vi "Get Channel Info.vi"(8 "error in (no error)":errorcluster, 11 "FPGA Personality File Path":path) -> (0 "error out":errorcluster, 2 "Channel Info":string[][](array[string]), 3 "Duplicated FPGA Personality File Path":path)   [LabVIEW 2021, in "Personality.lvlib"]
doc: "Gets all channal information from the specified FPGA personality file."
uses:
  <vilib>/myRIO/Common/FPGA Personality Framework/Personality.lvlib
  <vilib>/xml/Load XML File.vi
  <vilib>/xml/Close Reference(Node).vi
  <vilib>/xml/NI_XML.lvlib
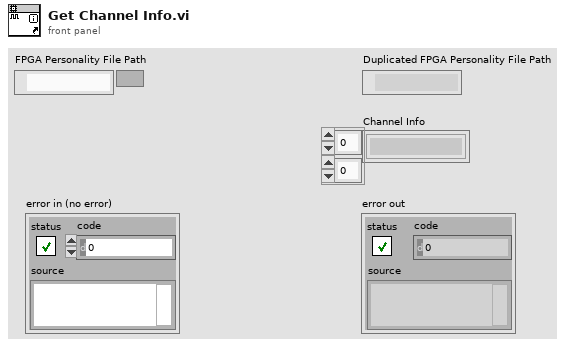
[diagram p1: front panel]
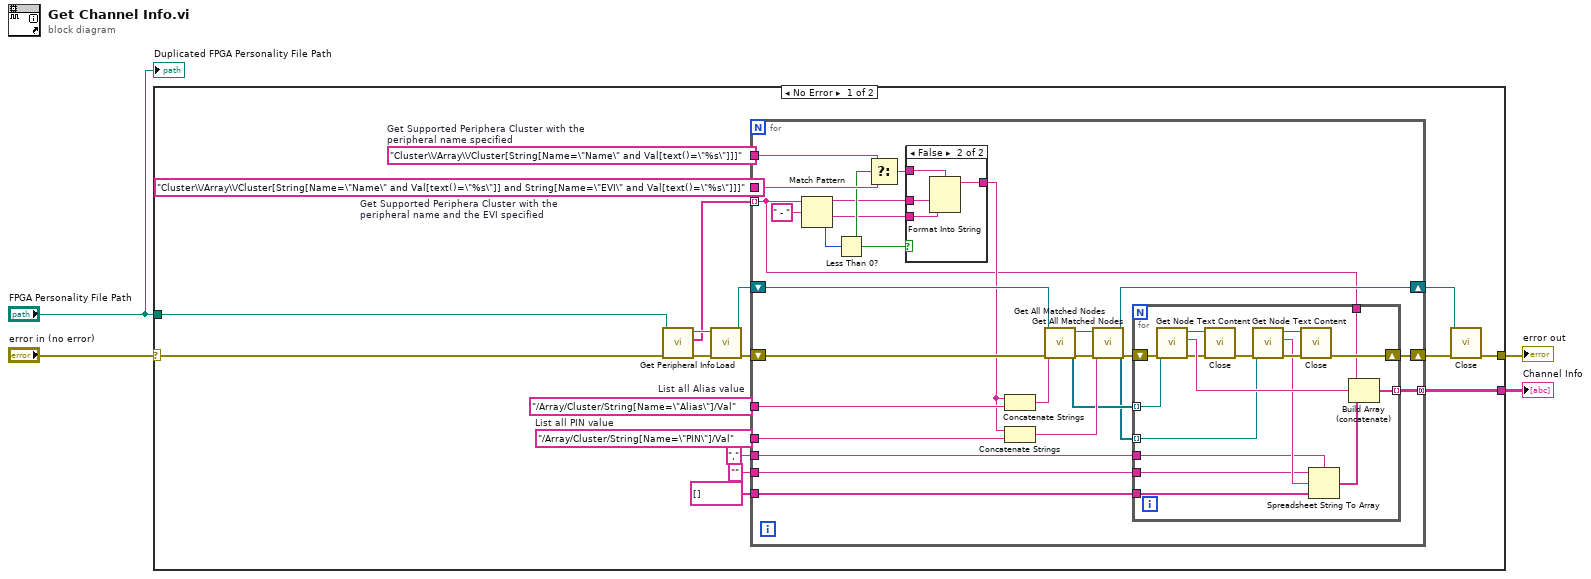
[diagram p0: block diagram]
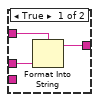
[diagram p2: hidden frame]
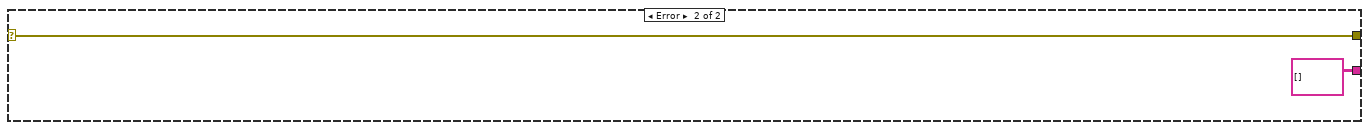
[diagram p3: hidden frame]
diagram:
  n1 = case shown="No Error" "error in (no error)" {
    selector: "error in (no error)" -> [w22 w75]
    tunnel: [w21 w75] -> w3
    tunnel: "FPGA Personality File Path" -> [w20 _]
    tunnel: [w5 string[][] []] -> w1
    frame No Error {
      w9 = "/Array/Cluster/String[Name=\"PIN\"]/Val"  # List all PIN value
      w10 = "/Array/Cluster/String[Name=\"Alias\"]/Val"  # List all Alias value
      w11 = "Cluster\\/Array\\/Cluster[String[Name=\"Name\" and Val[text()=\"%s\"]]]"  # Get Supported Periphera Cluster with the peripheral name specified
      w18 = "Cluster\\/Array\\/Cluster[String[Name=\"Name\" and Val[text()=\"%s\"]] and String[Name=\"EVI\" and Val[text()=\"%s\"]]]"  # Get Supported Periphera Cluster with the peripheral name and the EVI specified
      n2 = call <vilib>:"Get Peripheral Info.vi"("error in (no error)"=w22, "FPGA Personality File Path"=w20) -> ("error out"=w15:errorcluster, "Supported Peripherals"=w12:string[], "Duplicated FPGA Personality File Path"=w14:path)  [unwired: 6 in, 1 out]
      n3 = call-poly <vilib>:"Load.vi"("path to XML document"=w14, "error in (no error)"=w15) -> ("DOM document out"=w16:refnum<k20>, "error out"=w13:errorcluster)  [unwired: 11 in, 1 out]
      n4 = for {
        tunnel: w18 -> [w46]
        shift-right: [w25] -> w19
        shift-left: w13 -> [w49]
        shift-right: [w33] -> w17
        shift-left: w16 -> [w48]
        tunnel: w12 -> [w26] mode=indexing
        tunnel: w11 -> [w45]
        tunnel: w10 -> [w40]
        tunnel: w9 -> [w39]
        tunnel: "," ("delimiter (Tab)") -> [w29]
        tunnel: "" ("format string") -> [w28]
        tunnel: string[] [] -> [w27]
        tunnel: [w24] -> w5 mode=concatenating
        n5 = Match Pattern(string=w26, regular expression=" - ") -> (before substring=w42:string, after substring=w43:string, offset past match=w23:i32)  [unwired: 1 in, 1 out]
        n6 = Less Than 0?(x=w23) -> (x < 0?=w44:bool)
        n7 = Select(t=w45, s=w44, f=w46) -> (s? t:f=w41:string)
        n8 = case shown="False" w44 {
          tunnel: w43 -> [_ w70]
          tunnel: w42 -> [w68 w72]
          tunnel: w41 -> [w69 w73]
          tunnel: [w67 w71] -> w38
          frame True {
            n9 = Format Into String(format string=w69, w68) -> (resulting string=w67:string)  [unwired: 2 in, 1 out]
          }
          frame False {
            n10 = Format Into String(format string=w73, w72, w70) -> (resulting string=w71:string)  [unwired: 2 in, 1 out]
          }
        }
        n11 = Concatenate Strings(w38, w40) -> (w37:string)
        n12 = Concatenate Strings(w38, w39) -> (w36:string)
        n13 = call <vilib>:"Get All Matched Nodes.vi"("error in (no error)"=w49, "XPath expression"=w37, "node in"=w48) -> ("error out"=w34:errorcluster, "node result array"=w31:refnum<k20>[], "node out"=w35:refnum<k20>)  [unwired: 6 in]
        n14 = call <vilib>:"Get All Matched Nodes.vi"("error in (no error)"=w34, "XPath expression"=w36, "node in"=w35) -> ("error out"=w32:errorcluster, "node result array"=w30:refnum<k20>[], "node out"=w33:refnum<k20>)  [unwired: 6 in]
        n15 = for {
          shift-right: [w60] -> w25
          shift-left: w32 -> [w66]
          tunnel: [w65] -> w24 mode=indexing
          tunnel: w31 -> [w59] mode=indexing
          tunnel: w30 -> [w50] mode=indexing
          tunnel: w29 -> [w54]
          tunnel: w28 -> [w55]
          tunnel: w27 -> [w53]
          tunnel: w26 -> [w52]
          n16 = call <vilib>:"Get Node Text Content.vi"("error in (no error)"=w66, "node in"=w59) -> ("error out"=w62:errorcluster, "node text"=w63:string, "node out"=w58:refnum<k20>)  [unwired: 7 in]
          n17 = call-poly <vilib>:"Close.vi"("error in (no error)"=w62, "node"=w58) -> ("error out"=w61:errorcluster)  [unwired: 7 in]
          n18 = call <vilib>:"Get Node Text Content.vi"("error in (no error)"=w61, "node in"=w50) -> ("error out"=w64:errorcluster, "node text"=w56:string, "node out"=w57:refnum<k20>)  [unwired: 7 in]
          n19 = call-poly <vilib>:"Close.vi"("error in (no error)"=w64, "node"=w57) -> ("error out"=w60:errorcluster)  [unwired: 7 in]
          n20 = Spreadsheet String To Array(delimiter (Tab)=w54, format string=w55, spreadsheet string=w56, array type (2D Dbl)=w53) -> (array=w51:string[])
          n21 = Build Array (concatenate)(w52, w63, w51) -> (w65:string[])
        }
      }
      n22 = call-poly <vilib>:"Close.vi"("error in (no error)"=w19, "node"=w17) -> ("error out"=w21:errorcluster)  [unwired: 7 in]
    }
    frame Error {
    }
  }
  "Channel Info" <- w1
  "error out" <- w3
  "Duplicated FPGA Personality File Path" <- "FPGA Personality File Path"
